vi "Queue.vi"(8 "error in":errorcluster, 11 "Data":variant) -> (0 "Error out":errorcluster, 1 "Product name":string, 2 "UI Controllers":string[](array[string]), 3 "Enum":T2(ring), 4 "Module Number":dbl, 5 "Batch Data 3":T1)   [LabVIEW 2015, in "Copy of Untitled Library 1.lvlib"]
uses:
  Copy of Untitled Library 1.lvlib
  Controls/Caller Queue Control .ctl
  Controls/Control 1.ctl
panel:
  in  "Cluster":T3
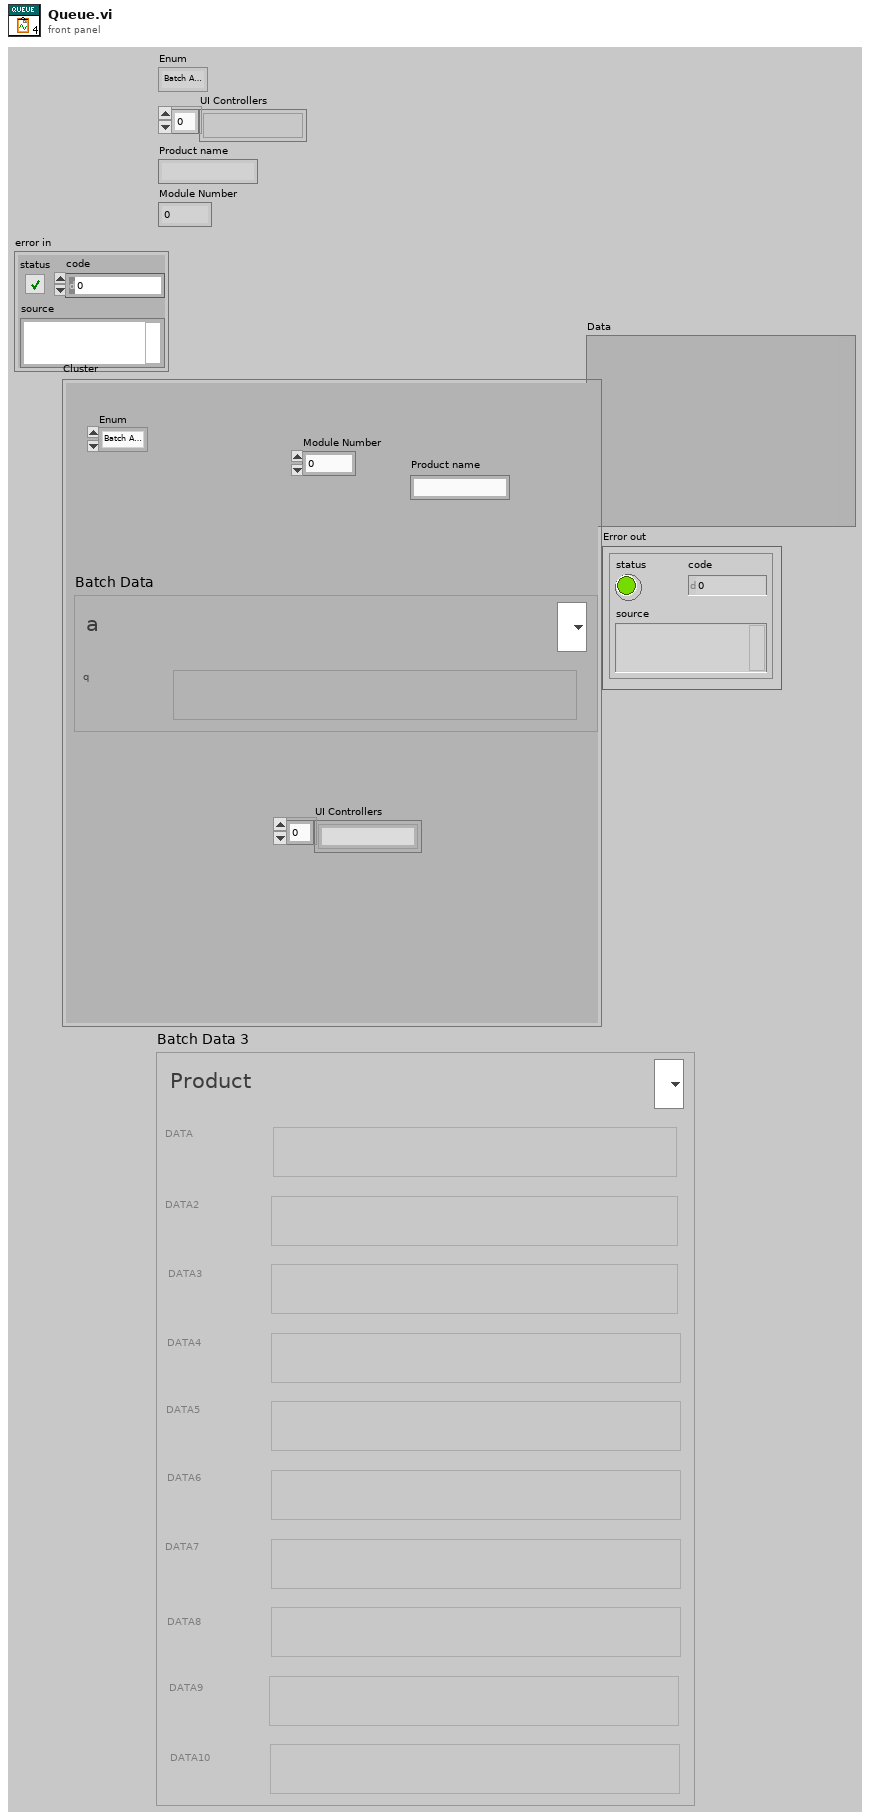
[diagram p1: front panel]
types:
  T1 = typedef "Copy of Untitled Library 1.lvlib/Control 1.ctl" = cluster{"DATA":string, "DATA 2":string, "DATA 3":string, "DATA 4":string, "DATA 5":string, "DATA 6":string, "DATA 7":string, "DATA 8":string, "DATA 9":string, "DATA 10":string, "Product":string}
  T2 = enum16{"Batch Added", "Batch Deleted", "Batch Opened", "Batch Closed", "Batch Edited", "new Product Added", "Product deleted "}
  T3 = typedef "Caller Queue Control .ctl" = cluster{"Enum":enum16{"Batch Added", "Batch Deleted", "Batch Opened", "Batch Closed", "Batch Edited", "new Product Added", "Product deleted "}, "Batch Data 3":T1, "UI Controllers":string[], "Product name":string, "Module Number":dbl}
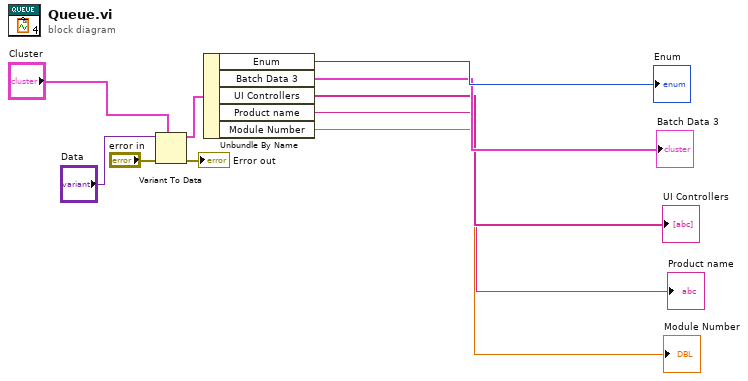
[diagram p0: block diagram]
diagram:
  n1 = Variant To Data(error in="error in", type="Cluster", Variant="Data") -> (data=w10:T3, error out=→"Error out":errorcluster)
  n2 = Unbundle By Name(w10) -> ("Enum"=→"Enum":T2, "Batch Data 3"=→"Batch Data 3":T1, "UI Controllers"=→"UI Controllers":string[], "Product name"=→"Product name":string, "Module Number"=→"Module Number":dbl)
